vi "niDTS BT LE Rx Test Get Default Limits.vi"(0 "Dummy Test Handle In":T2, 11 "error in (no error)":errorcluster) -> (4 "Dummy Test Handle Out":T2, 6 "USL":T1, 8 "LSL":T1, 15 "error out":errorcluster)   [LabVIEW 2014, in "niDTS BT.lvlib"]
uses:
  niDTS BT.lvlib
  BDR Tx Test/Includes/niDTS BT Rx Test INC Handle.ctl
  Rx Test/Objects/BASE_class/niDTS BT Rx Test.lvclass
  Rx Test/Includes/niDTS BT Rx Test INC Results.ctl
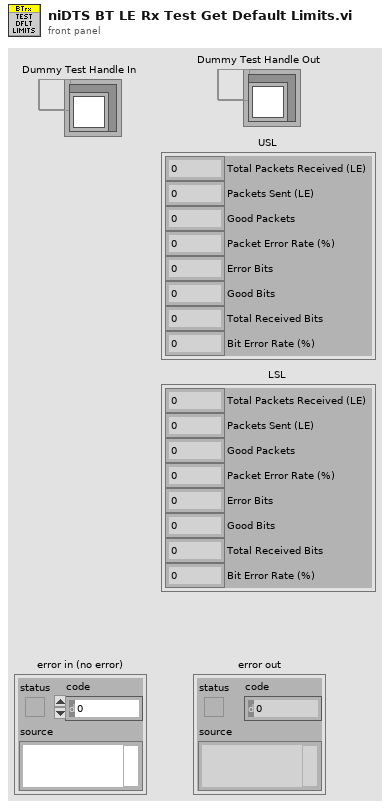
[diagram p1: front panel]
types:
  T1 = typedef "niDTS BT.lvlib/niDTS BT Rx Test INC Results.ctl" = cluster{"Total Packets Received (LE)":i32, "Packets Sent (LE)":dbl, "Good Packets":dbl, "Packet Error Rate (%)":dbl, "Error Bits":u32, "Good Bits":u32, "Total Received Bits":u32, "Bit Error Rate (%)":dbl}
  T2 = typedef "niDTS BT.lvlib/niDTS BT Rx Test INC Handle.ctl" = refnum<data-value>
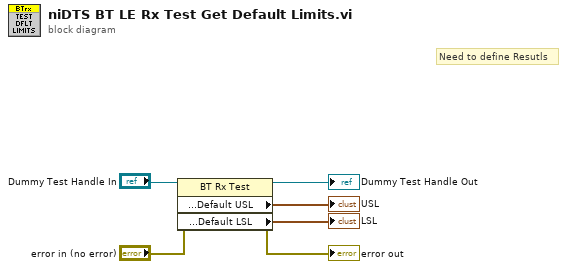
[diagram p0: block diagram]
diagram:
  # "Need to define Resutls"
  n1 = property class="BT Rx Test"(reference="Dummy Test Handle In", error in="error in (no error)") -> (reference out=→"Dummy Test Handle Out":T2, error out=→"error out":errorcluster, "Properties:Default Limits:Default USL"=→"USL":T1, "Properties:Default Limits:Default LSL"=→"LSL":T1)
